vi "getChannelArray.vi"(8 "error in (no error)":errorcluster, 11 "device.lvclass in":refnum<class "device.lvclass">) -> (0 "error out":errorcluster, 2 "ChannelArray.lvclass":refnum<class "ChannelArray.lvclass">, 3 "device.lvclass out":refnum<class "device.lvclass">)   [LabVIEW 2009, in "Tools.lvlib" / "DatabaseHelpers.lvlib" / "device.lvclass"]
uses:
  device.lvclass
  ChannelArray/ChannelArray.lvclass
  device.lvclass/device.ctl
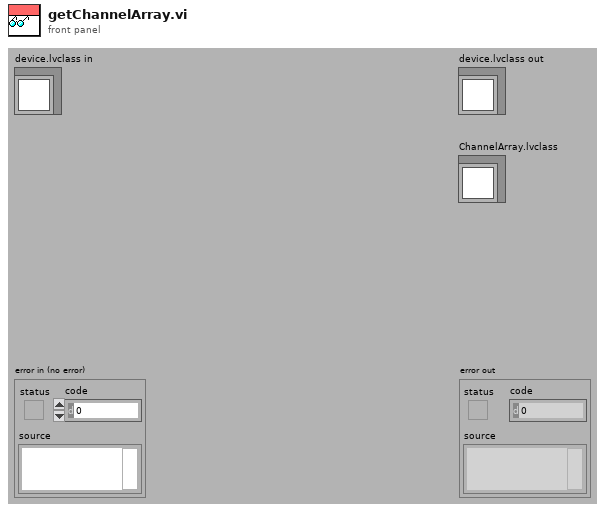
[diagram p1: front panel]
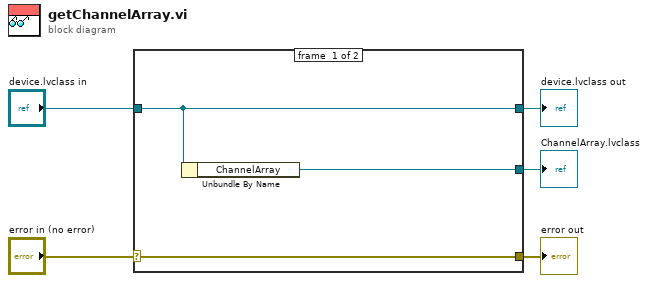
[diagram p0: block diagram]
diagram:
  n1 = case shown="No Error" "error in (no error)" {
    selector: "error in (no error)" -> [w8 w9]
    tunnel: [w8 w9] -> w4
    tunnel: [w7 w10] -> w2
    tunnel: "device.lvclass in" -> [w7 w10]
    tunnel: [w6 _] -> w1
    frame #0 {
      n2 = Unbundle By Name(w7) -> ("ChannelArray"=w6:refnum<class "ChannelArray.lvclass">)
    }
    frame #1 {
    }
  }
  "error out" <- w4
  "device.lvclass out" <- w2
  "ChannelArray.lvclass" <- w1
